vi "Z900_navX_Get_SystemInformation_Offsets.vi"(8 "error in (no error)":errorcluster, 11 "navX Device":T2={"Interface"={"Protocol"=enum."SERIAL", "Update Rate (4Hz-60Hz)"=4, "navX Open TypeDef"=variant}, "Notify Packet"=refnum, "Loop VI Refnum"=refnum, "Ready to Close Occurrence Refnum"=refnum} {"Interface"."Update Rate (4Hz-60Hz)" min=4 max=60 step=1}) -> (0 "error out":errorcluster, 1 "Connected":bool, 2 "Offsets":T1, 3 "navX Device":T2={"Interface"={"Protocol"=enum."SERIAL", "Update Rate (4Hz-60Hz)"=4, "navX Open TypeDef"=variant}, "Notify Packet"=refnum, "Loop VI Refnum"=refnum, "Ready to Close Occurrence Refnum"=refnum} {"Interface"."Update Rate (4Hz-60Hz)" min=4 max=60 step=1})   [LabVIEW 2015, in "navX Library v2.lvlib"]
doc: "This navX VI returns the Offsets of the navX. This VI is rarely needed."
uses:
  navX Library v2.lvlib
  TypeDefs/Z900_navX_DeviceTypeDef.ctl
  TypeDefs/Z900_navX_ProtocolTypeDef.ctl
  TypeDefs/Z900_navX_NotifyPacketTypeDef.ctl
  TypeDefs/Z900_navX_ActionTypeDef.ctl
  TypeDefs/Z900_navX_DeviceRegisters.ctl
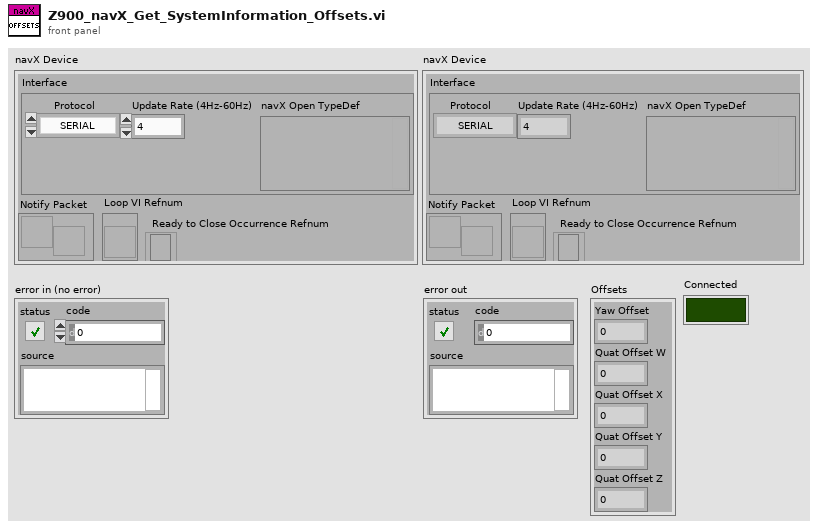
[diagram p1: front panel]
types:
  T1 = cluster{"Yaw Offset":dbl, "Quat Offset W":dbl, "Quat Offset X":dbl, "Quat Offset Y":dbl, "Quat Offset Z":dbl}
  T2 = typedef "navX Library v2.lvlib/Z900_navX_DeviceTypeDef.ctl" = cluster{"Interface":cluster{"Protocol":T3, "Update Rate (4Hz-60Hz)":u8, "navX Open TypeDef":variant}, "Notify Packet":refnum<notifier>, "Loop VI Refnum":refnum<vi>, "Ready to Close Occurrence Refnum":refnum<k4>}
  T3 = typedef "navX Library v2.lvlib/Z900_navX_ProtocolTypeDef.ctl" = enum16{"SERIAL", "I2C", "SPI"}
  T4 = typedef "navX Library v2.lvlib/Z900_navX_DeviceRegisters.ctl" = u8
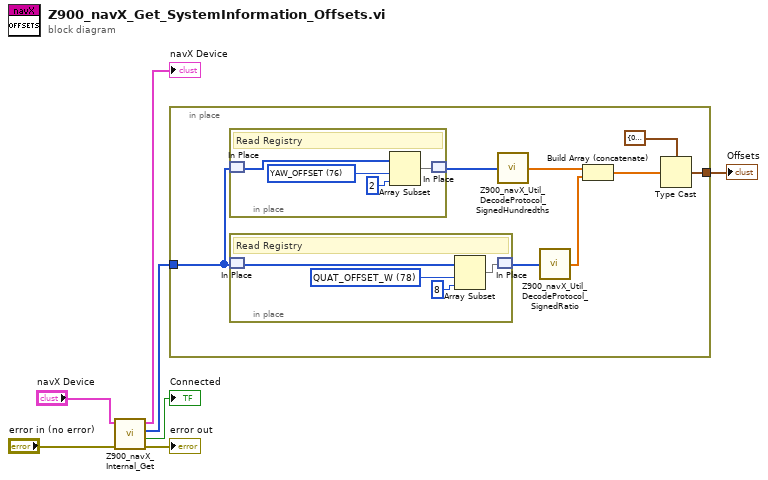
[diagram p0: block diagram]
diagram:
  n1 = call "Z900_navX_Internal_Get.vi"("error in (no error)"="error in (no error)", "navX Device"="navX Device") -> ("error out"=→"error out":errorcluster, "Connected"=→"Connected":bool, "Registry"=w3:u8[], "navX Device"=→"navX Device":T2)  [unwired: 6 in]
  n2 = in-place {
    in-place-border: w3 -> [w14]
    in-place-border: [w8] -> w2
    n3 = in-place {
      w22 = T4 76 items=["WHOAMI"=0, "HW_REV"=1, "FW_VER_MAJOR"=2, "FW_VER_MINOR"=3, "UPDATE_RATE_HZ"=4, "ACCEL_FSR_G"=5, "GYRO_FSR_DPS"=6, "OP_STATUS"=8, "CAL_STATUS"=9, "SELFTEST_STATUS"=10, "CAPABILITY_FLAGS_L"=11, "CAPABILITY_FLAGS_H"=12, "SENSOR_STATUS"=16, "TIMESTAMP"=18, "YAW"=22, "ROLL"=24, "PITCH"=26, "HEADING"=28, "FUSED_HEADING"=30, "ALTITUDE_I"=32, "ALTITUDE_D"=34, "LINERA_ACC_X"=36, "LINERA_ACC_Y"=38, "LINERA_ACC_Z"=40, "QUAT_W"=42, "QUAT_X"=44, "QUAT_Y"=46, "QUAT_Z"=48, "MPU_TEMP_C"=50, "GYRO_X"=52, "GYRO_Y"=54, "GYRO_Z"=56, "ACC_X"=58, "ACC_Y"=60, "ACC_Z"=62, "MAG_X"=64, "MAG_Y"=66, "MAG_Z"=68, "PRESSURE_I"=70, "PRESSURE_D"=72, "PRESSURE_TEMP"=74, "YAW_OFFSET"=76, "QUAT_OFFSET_W"=78, "QUAT_OFFSET_X"=80, "QUAT_OFFSET_Y"=82, "QUAT_OFFSET_Z"=84, "INTEGRATION_CONTROL"=86, "VELOCITY_X"=88, "VELOCITY_Y"=92, "VELOCITY_Z"=96, "DISPLACMENT_X"=100, "DISPLACMENT_Y"=104, "DISPLACEMENT_Z"=108] ("Device Register")
      # "Read Registry"
      n4 = in-place-match #1(w14) -> (w20:u8[])
      n5 = Array Subset(array=w20, index=w22, length=2) -> (w21:u8[])
      n6 = in-place-match #1(w21) -> (w15:u8[])
    }
    n7 = in-place {
      w18 = T4 78 items=["WHOAMI"=0, "HW_REV"=1, "FW_VER_MAJOR"=2, "FW_VER_MINOR"=3, "UPDATE_RATE_HZ"=4, "ACCEL_FSR_G"=5, "GYRO_FSR_DPS"=6, "OP_STATUS"=8, "CAL_STATUS"=9, "SELFTEST_STATUS"=10, "CAPABILITY_FLAGS_L"=11, "CAPABILITY_FLAGS_H"=12, "SENSOR_STATUS"=16, "TIMESTAMP"=18, "YAW"=22, "ROLL"=24, "PITCH"=26, "HEADING"=28, "FUSED_HEADING"=30, "ALTITUDE_I"=32, "ALTITUDE_D"=34, "LINERA_ACC_X"=36, "LINERA_ACC_Y"=38, "LINERA_ACC_Z"=40, "QUAT_W"=42, "QUAT_X"=44, "QUAT_Y"=46, "QUAT_Z"=48, "MPU_TEMP_C"=50, "GYRO_X"=52, "GYRO_Y"=54, "GYRO_Z"=56, "ACC_X"=58, "ACC_Y"=60, "ACC_Z"=62, "MAG_X"=64, "MAG_Y"=66, "MAG_Z"=68, "PRESSURE_I"=70, "PRESSURE_D"=72, "PRESSURE_TEMP"=74, "YAW_OFFSET"=76, "QUAT_OFFSET_W"=78, "QUAT_OFFSET_X"=80, "QUAT_OFFSET_Y"=82, "QUAT_OFFSET_Z"=84, "INTEGRATION_CONTROL"=86, "VELOCITY_X"=88, "VELOCITY_Y"=92, "VELOCITY_Z"=96, "DISPLACMENT_X"=100, "DISPLACMENT_Y"=104, "DISPLACEMENT_Z"=108] ("Device Register")
      # "Read Registry"
      n8 = in-place-match #2(w14) -> (w16:u8[])
      n9 = Array Subset(array=w16, index=w18, length=8) -> (w17:u8[])
      n10 = in-place-match #2(w17) -> (w13:u8[])
    }
    n11 = call "Z900_navX_Util_DecodeProtocol_SignedHundredths.vi"("Little Endian"=w15) -> ("Signed Hundredths (0.00)"=w12:dbl[])
    n12 = call "Z900_navX_Util_DecodeProtocol_SignedRatio.vi"("Little Endian"=w13) -> ("Signed Ratio"=w11:dbl[])
    n13 = Build Array (concatenate)(w12, w11) -> (w10:dbl[])
    n14 = Type Cast(type=T1 {"Yaw Offset"=0.0, "Quat Offset W"=0.0, "Quat Offset X"=0.0, "Quat Offset Y"=0.0, "Quat Offset Z"=0.0}, x=w10) -> (*(type *) &x=w8:T1)
  }
  "Offsets" <- w2
